vi "Read Data as Mono10 to Mono14 Packed Image.vi"(7 "n_bits":u8, 8 "error in (no error)":errorcluster, 11 "Buffer in":refnum<class "Buffer.lvclass">) -> (0 "error out":errorcluster, 2 "Image":u16[][](array[numeric]), 3 "Buffer":refnum<class "Buffer.lvclass">)   [LabVIEW 2020, in "Buffer.lvclass"]
uses:
  Buffer.lvclass
  Buffer.lvclass/Buffer.ctl
  bin/gindustrialcam_32-1.dll
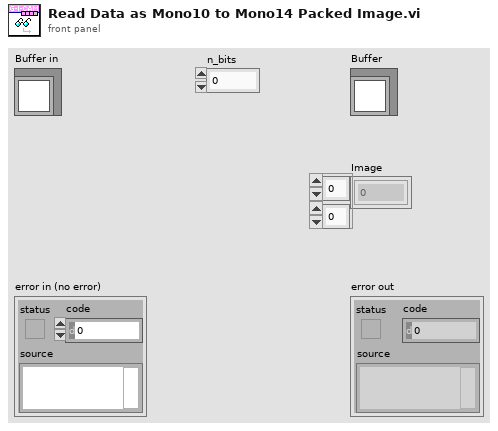
[diagram p1: front panel]
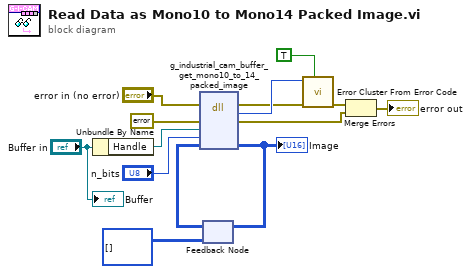
[diagram p0: block diagram]
diagram:
  n1 = Unbundle By Name("Buffer in") -> ("Handle"=w2:refnum<data-value>)
  n2 = feedback #1(u16[][] [] ("Image")) -> (w4:u16[][])
  n3 = dll-call lib="C:/serenial/lib/g-industrial-camera/LabVIEW/g_industrial_cam/bin/gindustrialcam_*-1.*" fn="g_industrial_cam_buffer_get_mono10_to_14_packed_image"(error in="error in (no error)", "err"=errorcluster {"status"=FALSE, "code"=0, "source"=""} ("error constant"), "edvr"=w2, "n_bits"="n_bits", "Image"=w4) -> (error out=w8:errorcluster, "Mg_Error"=w9:i32, "err"=w11:errorcluster, "Image"=w5:u16[][])  [unwired: 4 in, 1 out]
  "Image" <- w5
  n4 = feedback-in #1(w5) -> ()
  n5 = call <vilib>:"Error Cluster From Error Code.vi"("show call chain? (False)"=TRUE, "error in (no error)"=w8, "error code (0)"=w9) -> ("error out"=w10:errorcluster)  [unwired: 6 in]
  n6 = Merge Errors(w10, w11) -> (→"error out":errorcluster)
  "Buffer" <- "Buffer in"
